vi "Queue.vi"(7 "State":T1, 8 "error in":errorcluster caption="错误输入", 10 "Data":variant[](array[variant]), 11 "Instruct":string[](array[string])) -> (0 "error out":errorcluster caption="错误输出", 2 "Data Out":variant, 3 "Instruct Out":string)   [LabVIEW 2020]
uses:
  Control/QueueState.ctl
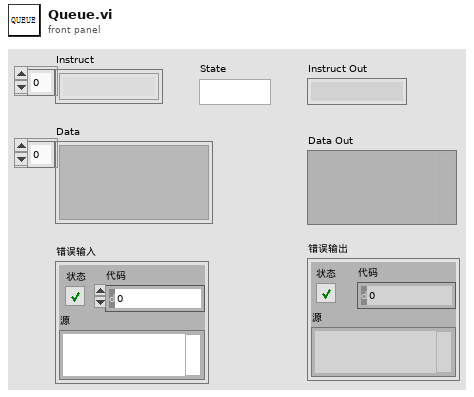
[diagram p1: front panel]
types:
  T1 = typedef "QueueState.ctl" = enum16{"", "Create", "In", "Out", "Empty", "Close"}
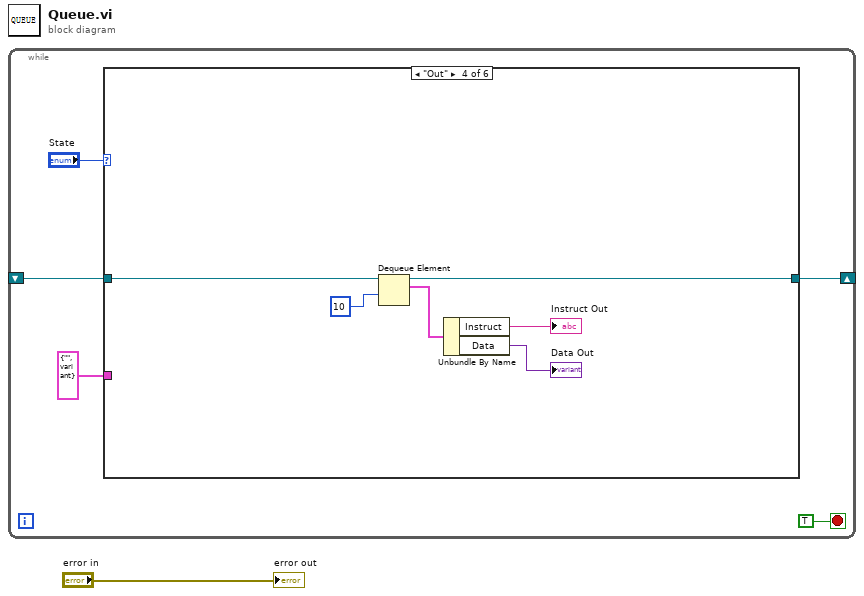
[diagram p0: block diagram]
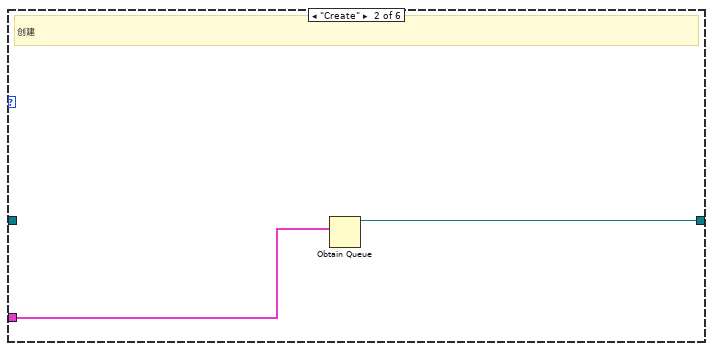
[diagram p3: hidden frame]
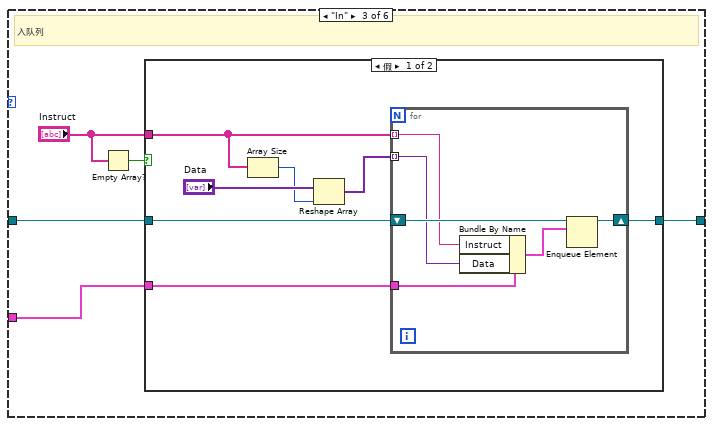
[diagram p4: hidden frame]
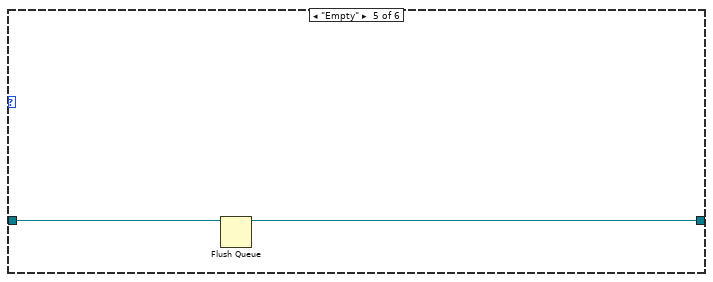
[diagram p6: hidden frame]
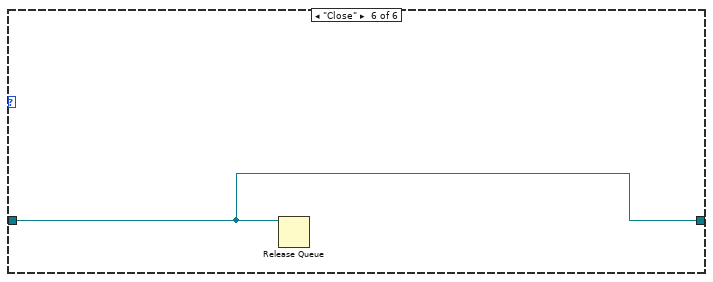
[diagram p7: hidden frame]
diagram:
  n1 = while {
    shift-right: [w3] -> _
    shift-left: _ -> [w2]
    stop <- TRUE stop-if-true
    n2 = case shown="\"Out\"" "State" {
      tunnel: cluster{"Instruct":string, "Data":variant} {"Instruct"="", "Data"=variant} -> [_ w9 w13 _ _ _]
      tunnel: [w7 w8 w12 w33 w35 w37] -> w3
      tunnel: w2 -> [w7 _ w14 w34 w36 w37]
      frame "", Default {
      }
      frame "Create" {
        # "创建"
        n3 = Obtain Queue(element data type=w9) -> (queue out=w8:refnum<queue>)  [unwired: 4 in, 2 out]
      }
      frame "In" {
        # "入队列"
        n4 = Empty Array?(array="Instruct") -> (empty?=w11:bool)
        n5 = case shown="假" w11 {
          tunnel: "Instruct" -> [w19 _]
          tunnel: w14 -> [w17 w28]
          tunnel: w13 -> [w16 _]
          tunnel: [w15 w28] -> w12
          frame False {
            n6 = Array Size(array=w19) -> (size(s)=w20:i32)
            n7 = Reshape Array("Data", w20) -> (w18:variant[])
            n8 = for {
              tunnel: w19 -> [w24] mode=indexing
              tunnel: w18 -> [w23] mode=indexing
              shift-right: [w26] -> w15
              shift-left: w17 -> [w27]
              tunnel: w16 -> [w25]
              n9 = Bundle By Name(cluster=w25, "Instruct"=w24, "Data"=w23) -> (w22:cluster{"Instruct":string, "Data":variant})
              n10 = Enqueue Element(queue=w27, element=w22) -> (queue out=w26:refnum<queue>)  [unwired: 2 in, 2 out]
            }
          }
          frame True {
          }
        }
      }
      frame "Out" {
        n11 = Dequeue Element(queue=w34, timeout in ms (-1)=10 ("超时毫秒(-1)")) -> (queue out=w33:refnum<queue>, element=w31:cluster{"Instruct":string, "Data":variant})  [unwired: 1 in, 2 out]
        n12 = Unbundle By Name(w31) -> ("Instruct"=→"Instruct Out":string, "Data"=→"Data Out":variant)
      }
      frame "Empty" {
        n13 = Flush Queue(queue=w36) -> (queue out=w35:refnum<queue>)  [unwired: 1 in, 2 out]
      }
      frame "Close" {
        n14 = Release Queue(queue=w37) -> ()  [unwired: 2 in, 3 out]
      }
    }
  }
  "error out" <- "error in"
